vi "GenerateWaveform.vi"(1 "FMInfo":T1={"buffer size"=0, "bits"=0, "CarrierInfo"={"frequency"=10.0, "amplitude"=1.0, "sample rate"=0, "waveform type"=enum."Sine"}, "ModulatorInfo"={"frequency"=10.0, "amplitude"=1.0, "sample rate"=0, "waveform type"=enum."Sine"}, "Feedback"=FALSE} {"ModulatorInfo"."amplitude" format="%0.2p"; "ModulatorInfo"."frequency" format="%0.2p"; "CarrierInfo"."amplitude" format="%0.2p"; "CarrierInfo"."frequency" format="%0.2p"}) -> (0 "generated signal":dbl[](array[numeric]))   [LabVIEW 2016]
uses:
  GenerateWaveform/FMInfo.ctl
  Oscillator/WaveformType.ctl
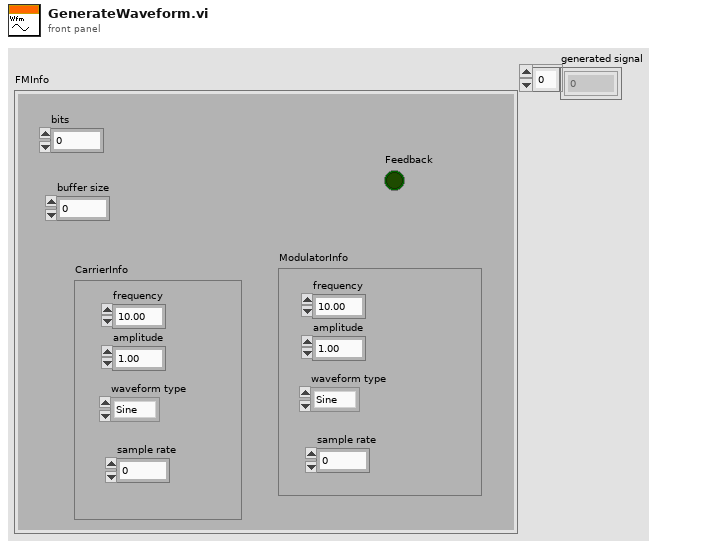
[diagram p1: front panel]
types:
  T1 = typedef "FMInfo.ctl" = cluster{"buffer size":i32, "bits":i32, "CarrierInfo":cluster{"frequency":dbl, "amplitude":dbl, "sample rate":i32, "waveform type":T2}, "ModulatorInfo":cluster{"frequency":dbl, "amplitude":dbl, "sample rate":i32, "waveform type":T2}, "Feedback":bool}
  T2 = typedef "WaveformType.ctl" = enum16{"Sine", "Triangle", "Square", "Sawtooth"}
  T3 = cluster{"frequency":dbl, "amplitude":dbl, "sample rate":i32, "waveform type":T2}
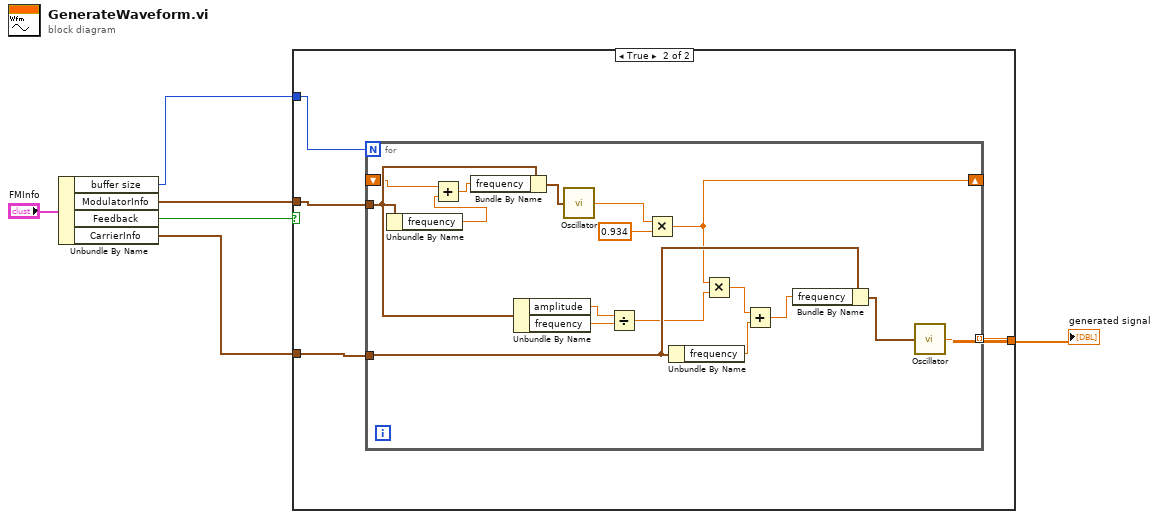
[diagram p0: block diagram]
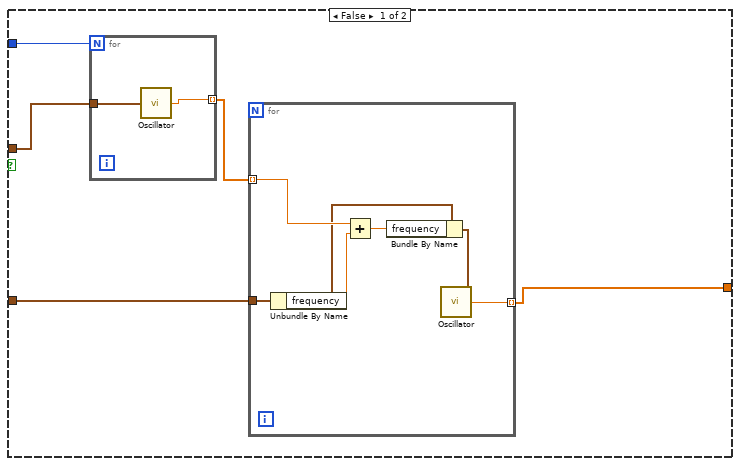
[diagram p2: hidden frame]
diagram:
  n1 = Unbundle By Name("FMInfo") -> ("buffer size"=w5:i32, "ModulatorInfo"=w1:T3, "Feedback"=w2:bool, "CarrierInfo"=w3:T3)
  n2 = case shown="True" w2 {
    tunnel: w1 -> [w10 w21]
    tunnel: w3 -> [w9 w22]
    tunnel: w5 -> [w8 w23]
    tunnel: [w7 w20] -> w4
    frame False {
      n3 = for {
        N: w8 -> [_]
        tunnel: [w12] -> w11 mode=indexing
        tunnel: w10 -> [w13]
        n4 = call "Oscillator.vi"("OscillatorInfo"=w13) -> ("output sample"=w12:dbl)
      }
      n5 = for {
        tunnel: w11 -> [w19] mode=indexing
        tunnel: w9 -> [w17]
        tunnel: [w18] -> w7 mode=indexing
        n6 = Unbundle By Name(w17) -> ("frequency"=w15:dbl)
        n7 = Add(x=w19, y=w15) -> (x+y=w16:dbl)
        n8 = Bundle By Name(cluster=w17, "frequency"=w16) -> (w14:T3)
        n9 = call "Oscillator.vi"("OscillatorInfo"=w14) -> ("output sample"=w18:dbl)
      }
    }
    frame True {
      n10 = for {
        N: w23 -> [_]
        tunnel: w22 -> [w40]
        tunnel: w21 -> [w33]
        tunnel: [w28] -> w20 mode=indexing
        shift-right: [w27] -> _
        shift-left: _ -> [w26]
        n11 = Unbundle By Name(w33) -> ("frequency"=w30:dbl)
        n12 = Add(x=w26, y=w30) -> (x+y=w29:dbl)
        n13 = Bundle By Name(cluster=w33, "frequency"=w29) -> (w32:T3)
        n14 = Unbundle By Name(w33) -> ("amplitude"=w35:dbl, "frequency"=w34:dbl)
        n15 = call "Oscillator.vi"("OscillatorInfo"=w32) -> ("output sample"=w31:dbl)
        n16 = Divide(x=w35, y=w34) -> (x/y=w25:dbl)
        n17 = Multiply(x=w31, y=0.934) -> (x*y=w27:dbl)
        n18 = Unbundle By Name(w40) -> ("frequency"=w38:dbl)
        n19 = Multiply(x=w27, y=w25) -> (x*y=w36:dbl)
        n20 = Add(x=w36, y=w38) -> (x+y=w37:dbl)
        n21 = Bundle By Name(cluster=w40, "frequency"=w37) -> (w39:T3)
        n22 = call "Oscillator.vi"("OscillatorInfo"=w39) -> ("output sample"=w28:dbl)
      }
    }
  }
  "generated signal" <- w4
